vi "GetEvtSignal.vi"(8 "error in (no error)":errorcluster, 11 "C37EventPlugin in":refnum<class "UserWfrmPlugins.lvclass">) -> (0 "error out":errorcluster, 3 "C37EventPlugin out":refnum<class "UserWfrmPlugins.lvclass">)   [LabVIEW 2014, in "WfrmPlugins.lvlib" / "UserWfrmPlugins.lvclass"]
uses:
  UserWfrmPlugins.lvclass
  <vilib>/Utility/config.llb/Read Key (String).vi
  <vilib>/imath/engines/lvmath/Plug In/_Char/NIMS_CH_String to Character Array.vi
  <vilib>/imath/engines/lvmath2/RunTimeEngine/IndexRead/NIMS V(S).vi
  <instcachedir>/0/NIMS V(S)_0488751826AF41519A22953C041130DC.lvgen/NIMS V(S)_0488751826AF41519A22953C041130DC_000.vi
  <vilib>/imathl/engines/lvmath/Functions/Error Handling/Create Error.vi
  <vilib>/imath/engines/lvmath2/RunTimeEngine/RangeToken/NIMS_Range.vi
  <instcachedir>/0/NIMS_Range_9BCE657718DF4976A877346C61F22738.lvgen/NIMS_Range_9BCE657718DF4976A877346C61F22738_000.vi
  C:/Labview Data/MathScriptVIs/MCStatic_33564263232_af0cd013292a3e2d5512c6b2b326fae0.vi
  <instcachedir>/0/MCStatic_33564263232_af0cd013292a3e2d5512c6b2b326fae0_3B518BEA2B9C45CB8A1676855454D908.lvgen/MCStatic_33564263232_af0cd013292a3e2d5512c6b2b326fae0_3B518BEA2B9C45CB8A1676855454D908_000.vi
  <vilib>/imath/engines/lvmath2/RunTimeEngine/UserFunctionToken/NIMS_UserFunction_CondDefined.vi
  <instcachedir>/0/NIMS_UserFunction_CondDefined_359D6D699583402F98E5D4DB7FB40D41.lvgen/NIMS_UserFunction_CondDefined_359D6D699583402F98E5D4DB7FB40D41_002.vi
  <vilib>/imath/engines/lvmath2/RunTimeEngine/VariableToken/NIMS_VariableToken_CondDefined.vi
  <instcachedir>/0/NIMS_VariableToken_CondDefined_EE8DD211A89249938CE6537267F5C9B3.lvgen/NIMS_VariableToken_CondDefined_EE8DD211A89249938CE6537267F5C9B3_001.vi
  <vilib>/imath/engines/lvmath2/RunTimeEngine/NodeEndStatement/NIMS_NodeEndStatement_Output.vi
  <instcachedir>/0/NIMS_NodeEndStatement_Output_53EC0D466D134D7ABD903AC30B43404B.lvgen/NIMS_NodeEndStatement_Output_53EC0D466D134D7ABD903AC30B43404B_002.vi
  <vilib>/imath/engines/lvmath2/RunTimeEngine/ErrorHandling/NIMS_Finalize Error.vi
  Matlab/User/UserEvtSigWrapper.m
  Matlab/User/Harm60255Sig.m
  <vilib>/Utility/config.llb/NI_LVConfig.lvlib
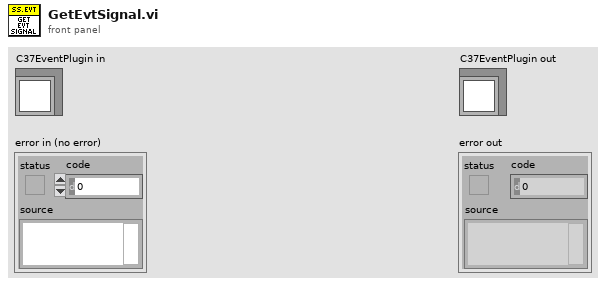
[diagram p1: front panel]
types:
  T1 = typedef "WfrmPlugins.lvlib/BaseWfrmPlugin.lvclass/WfrmConfig.ctl" = cluster{"T0(UTC)":dbl, "F0":dbl, "Fs":i32, "FSamp":u32}
  T2 = typedef "NI_LVConfig.lvlib/Config Data RefNum.ctl" = refnum<k1>
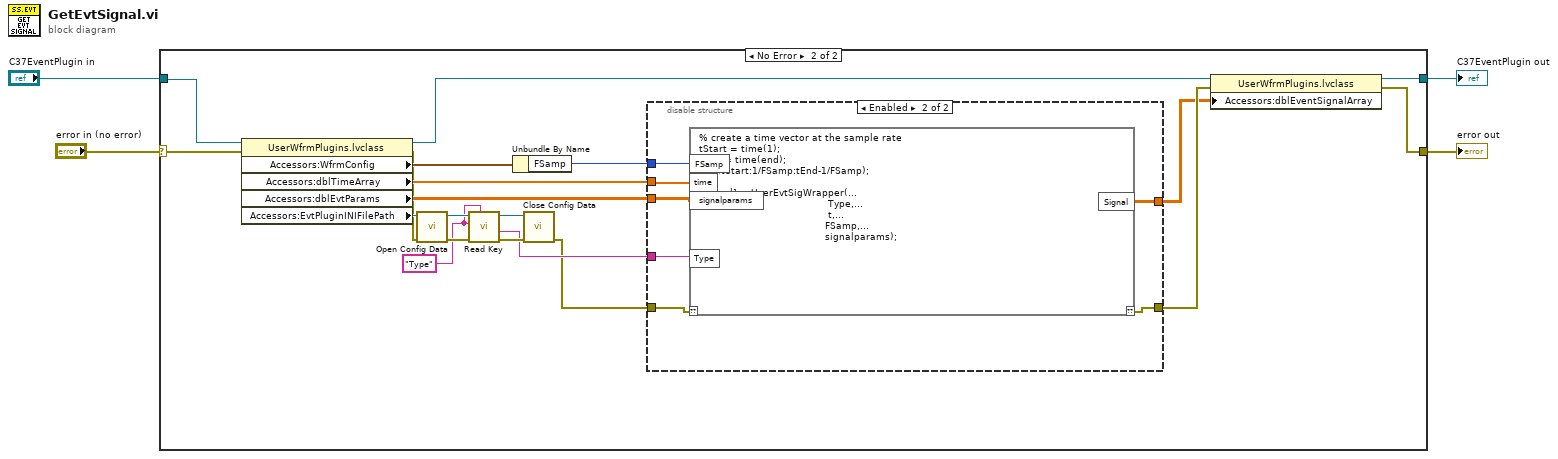
[diagram p0: block diagram]
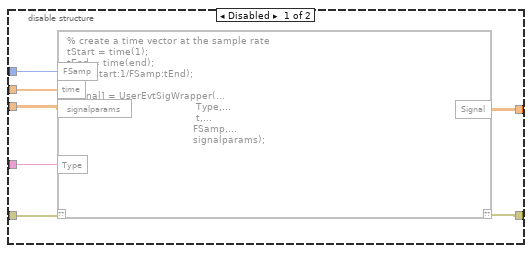
[diagram p3: hidden frame]
diagram:
  n1 = case shown="No Error" "error in (no error)" {
    selector: "error in (no error)" -> [w6 w23]
    tunnel: [w5 w26] -> w4
    tunnel: "C37EventPlugin in" -> [w5 w24]
    tunnel: [w6 w25] -> w3
    frame Error {
    }
    frame No Error {
      w11 = "Type" ("section")
      n2 = property class="UserWfrmPlugins.lvclass"(reference=w24, error in=w23) -> (reference out=w20:refnum<class "UserWfrmPlugins.lvclass">, error out=w14:errorcluster, "Accessors:WfrmConfig"=w22:T1, "Accessors:dblTimeArray"=w18:dbl[], "Accessors:dblEvtParams"=w17:dbl[][], "Accessors:EvtPluginINIFilePath"=w15:path)
      n3 = call <vilib>:"Open Config Data.vi"("error in (no error)"=w14, "configuration file path"=w15) -> ("error out"=w13:errorcluster, "refnum"=w12:T2)  [unwired: 7 in, 1 out]
      n4 = call-poly <vilib>:"Read Key.vi"("section"=w11, "error in (no error)"=w13, "key"=w11, "refnum"=w12) -> ("error out"=w10:errorcluster, "value"=w8:string, "refnum out"=w9:T2)  [unwired: 4 in, 1 out]
      n5 = Unbundle By Name(w22) -> ("FSamp"=w21:u32)
      n6 = call <vilib>:"Close Config Data.vi"("error in (no error)"=w10, "refnum"=w9) -> ("error out"=w7:errorcluster)  [unwired: 8 in, 1 out]
      n7 = disable-structure shown="Enabled" {
        disable-tunnel: w21 -> [w33 w38]
        disable-tunnel: [w32 w39] -> w19
        disable-tunnel: w18 -> [w31 w37]
        disable-tunnel: w17 -> [w30 w36]
        disable-tunnel: [w29 w34] -> w16
        disable-tunnel: w8 -> [w28 w35]
        disable-tunnel: w7 -> [w27 w40]
        frame Disabled {
          n8 = script code="% create a time vector at the sample rate\ntStart = time(1);\ntEnd = time(end);\nt = (tStart:1/FSamp:tEnd);\n\n[Signal] = UserEvtSigWrapper(...\n                                           Type,...\n                                           t,...\n                                          FSamp,...\n                                          signalparams);"("??"=w27, "FSamp"=w33, "time"=w31, "signalparams"=w30, "Type"=w28) -> ("??"=w32:errorcluster, "Signal"=w29:dbl[][])
        }
        frame Enabled {
          n9 = mathscript code="% create a time vector at the sample rate\ntStart = time(1);\ntEnd = time(end);\nt = (tStart:1/FSamp:tEnd-1/FSamp);\n\n[Signal] = UserEvtSigWrapper(...\n                                           Type,...\n                                           t,...\n                                          FSamp,...\n                                          signalparams);"("??"=w40, "FSamp"=w38, "time"=w37, "signalparams"=w36, "Type"=w35) -> ("??"=w39:errorcluster, "Signal"=w34:dbl[][])
        }
      }
      n10 = property class="UserWfrmPlugins.lvclass"(reference=w20, error in=w19, "Accessors:dblEventSignalArray"=w16) -> (reference out=w26:refnum<class "UserWfrmPlugins.lvclass">, error out=w25:errorcluster)
    }
  }
  "error out" <- w3
  "C37EventPlugin out" <- w4
